vi "Logging AddEdit Tree Item.vi"(2 "Log Entry":T1, 3 "TreeRef":refnum<vi>) -> (1 "TreeRef":refnum<vi>)   [LabVIEW 2012, in "femtoRoboLib.lvlib"]
uses:
  Controls/Log Entry.ctl
  Controls/Log Value Type.ctl
  Controls/Log Value Cluster.ctl
  femtoRoboLib.lvlib
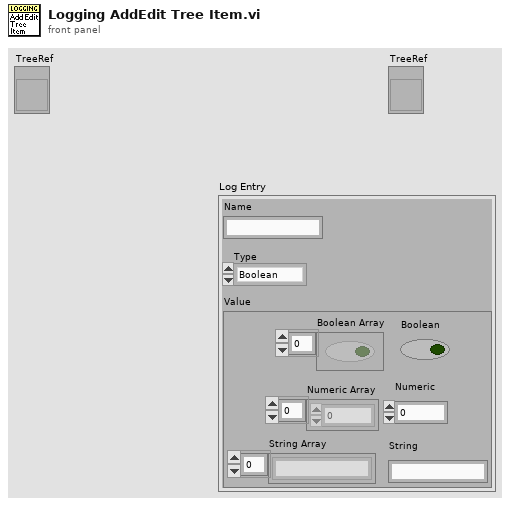
[diagram p1: front panel]
types:
  T1 = typedef "femtoRoboLib.lvlib/Log Entry.ctl" = cluster{"Name":string, "Type":T2, "Value":T3}
  T2 = typedef "femtoRoboLib.lvlib/Log Value Type.ctl" = enum16{"Boolean", "Numeric", "String", "Boolean Array", "Numeric Array", "String Array"}
  T3 = typedef "femtoRoboLib.lvlib/Log Value Cluster.ctl" = cluster{"Boolean Array":bool[], "Boolean":bool, "Numeric Array":dbl[], "Numeric":dbl, "String Array":string[], "String":string}
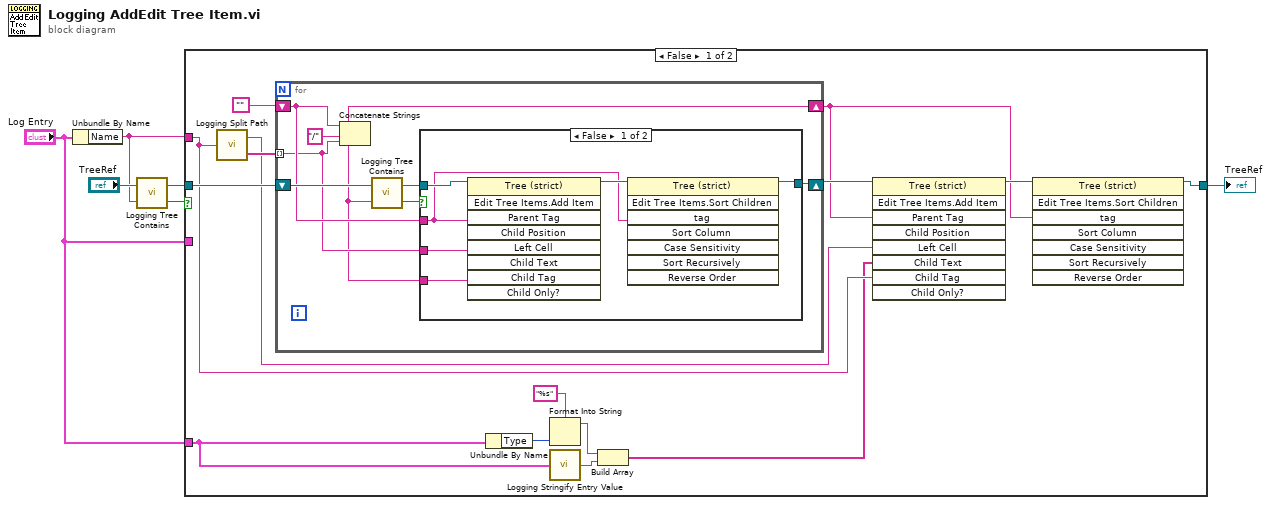
[diagram p0: block diagram]
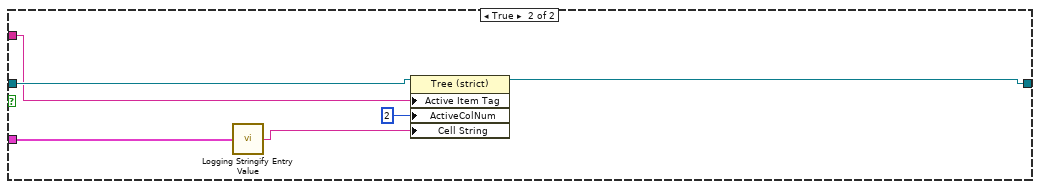
[diagram p3: hidden frame]
diagram:
  n1 = Unbundle By Name("Log Entry") -> ("Name"=w2:string)
  n2 = call "Logging Tree Contains.vi"("Name"=w2, "TreeRef"="TreeRef") -> ("Contained"=w4:bool, "TreeRef"=w5:refnum<vi>)
  n3 = case shown="False" w4 {
    tunnel: w5 -> [w19 w40]
    tunnel: w2 -> [w14 w39]
    tunnel: [w16 w41] -> w3
    tunnel: "Log Entry" -> [w8 _]
    tunnel: "Log Entry" -> [_ w37]
    frame False {
      n4 = call "Logging Split Path.vi"("Path In"=w14) -> ("Name"=w13:string, "Split Path"=w21:string[])
      n5 = for {
        tunnel: w21 -> [w24] mode=indexing
        shift-right: [w23] -> w15
        shift-left: "" -> [w26]
        shift-right: [w22] -> w18
        shift-left: w19 -> [w29]
        n6 = Concatenate Strings(w26, "/", w24) -> (w23:string)
        n7 = call "Logging Tree Contains.vi"("Name"=w23, "TreeRef"=w29) -> ("Contained"=w27:bool, "TreeRef"=w25:refnum<vi>)
        n8 = case shown="False" w27 {
          tunnel: w26 -> [w31 _]
          tunnel: w25 -> [w35 w36]
          tunnel: w24 -> [w34 _]
          tunnel: w23 -> [w33 _]
          tunnel: [w30 w36] -> w22
          frame False {
            n9 = invoke class="Tree (strict)" method="Edit Tree Items.Add Item"(reference=w35, "Parent Tag"=w31, "Left Cell"=w34, "Child Tag"=w33) -> (reference out=w32:refnum<vi>)  [unwired: 5 in, 8 out]
            n10 = invoke class="Tree (strict)" method="Edit Tree Items.Sort Children"(reference=w32, "tag"=w31) -> (reference out=w30:refnum<vi>)  [unwired: 6 in, 7 out]
          }
          frame True {
          }
        }
      }
      n11 = Unbundle By Name(w8) -> ("Type"=w11:T2)
      n12 = Format Into String(format string="%s", w11) -> (resulting string=w10:string)  [unwired: 2 in, 1 out]
      n13 = call "Logging Stringify Entry Value.vi"("Entry"=w8) -> ("String"=w9:string)
      n14 = Build Array(w10, w9) -> (w7:string[])
      n15 = invoke class="Tree (strict)" method="Edit Tree Items.Add Item"(reference=w18, "Parent Tag"=w15, "Left Cell"=w13, "Child Text"=w7, "Child Tag"=w14) -> (reference out=w17:refnum<vi>)  [unwired: 4 in, 8 out]
      n16 = invoke class="Tree (strict)" method="Edit Tree Items.Sort Children"(reference=w17, "tag"=w15) -> (reference out=w16:refnum<vi>)  [unwired: 6 in, 7 out]
    }
    frame True {
      n17 = call "Logging Stringify Entry Value.vi"("Entry"=w37) -> ("String"=w38:string)
      n18 = property class="Tree (strict)"(reference=w40, "Active Item Tag"=w39, "ActiveColNum"=2 ("Active Cell:Active Column Number"), "Cell String"=w38) -> (reference out=w41:refnum<vi>)  [unwired: 1 in, 1 out]
    }
  }
  "TreeRef" <- w3
